vi "ImageNorm.vi"(1 "Numeric":i32, 2 "Array":dbl[][][](array[numeric])) -> (0 "Fractional Change 2":dbl[][](graph))   [LabVIEW 2009]
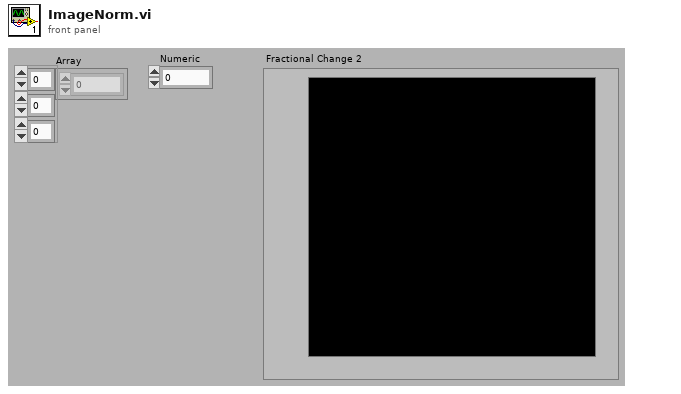
[diagram p1: front panel]
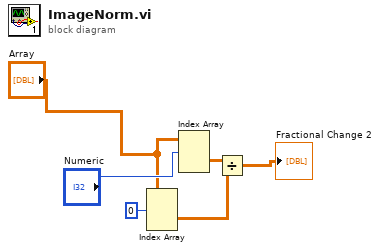
[diagram p0: block diagram]
diagram:
  n1 = Index Array(array="Array", index (dim 0)=0 ("index (page)")) -> (element=w2:dbl[][])  [unwired: 2 in]
  n2 = Index Array(array="Array", index (dim 0)="Numeric") -> (element=w3:dbl[][])  [unwired: 2 in]
  n3 = Divide(x=w3, y=w2) -> (x/y=→"Fractional Change 2":dbl[][])
